vi "Recast Device.vi"(8 "error in":errorcluster, 11 "AlicatCommBank in":refnum<class "AlicatCommBank.lvclass">) -> (0 "error out":errorcluster, 3 "AlicatCommBank out":refnum<class "AlicatCommBank.lvclass">)   [LabVIEW 2015, in "Alicat.lvlib" / "AlicatCommBank.lvclass"]
doc: "This VI takes the Model number data and uses it to correctly cast the device types. Use this in conjunction with the Read Models VI to ensure that the model numbers are properly read in first. \n\nAlso, check register 20 - if the value is greater than 32768, then the controller is set up for back pressure control. In this case, we do not want to use the manufacturing data (since that will only tell the program the FS flow rate). Rather, use the original programatic input. If the input at config time is not correct, then the output will not scale correctly."
uses:
  AlicatCommBank.lvclass
  AlicatCommBank.lvclass/AlicatCommBank.ctl
  M/M.lvclass
  VC/Alicat_VC.lvclass
  V/V.lvclass
  P/P.lvclass
  MC/Alicat_MC.lvclass
  Alicat.lvclass
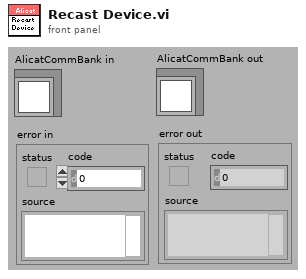
[diagram p1: front panel]
types:
  T1 = typedef "Alicat.lvlib/Alicat.lvclass/CtlSetup.ctl" = cluster{"Name":string, "Address":string, "fullScale":dbl, "Gas":T2}
  T2 = typedef "Alicat.lvlib/Alicat.lvclass/Gas.ctl" = enum16{"Air", "Ar", "CH4", "CO", "CO2", "C2H6", "H2", "He", "N2", "NO", "Ne", "O2", "C3H8", "n-C4H10", "C2H2", "C2H4", "i-C2H10", "Kr", "Xe"}
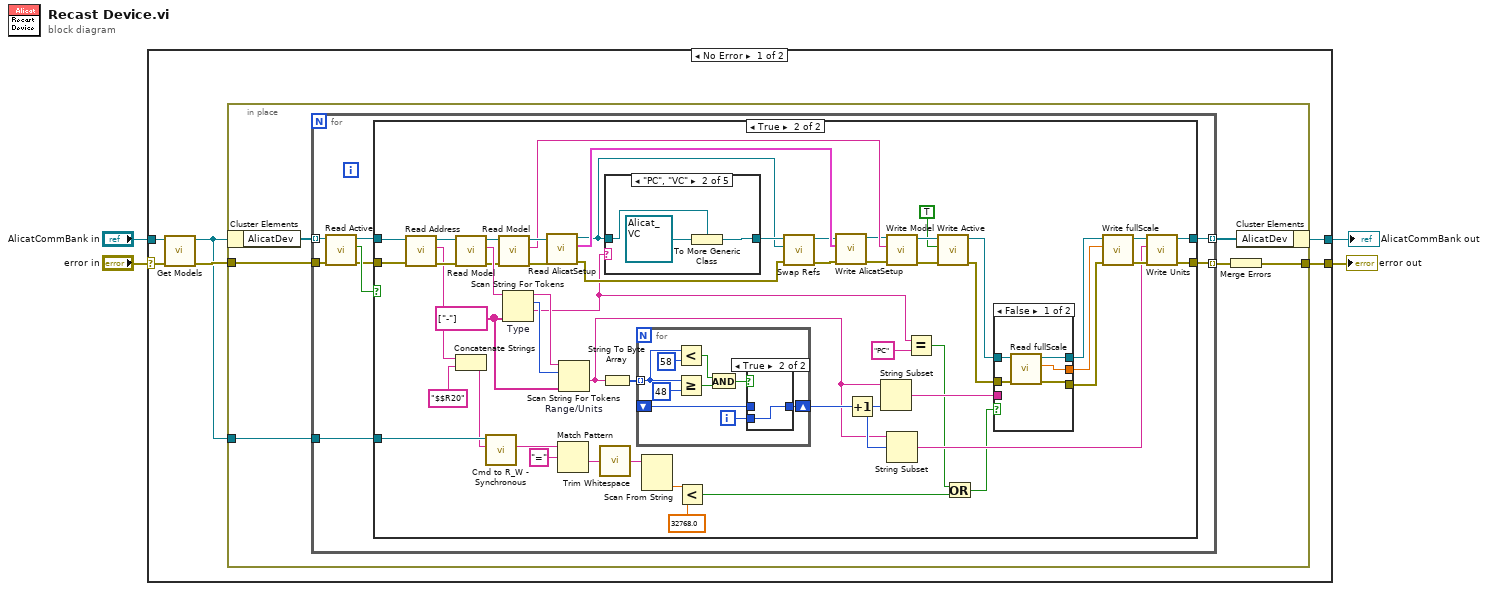
[diagram p0: block diagram]
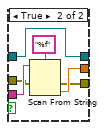
[diagram p3: hidden frame]
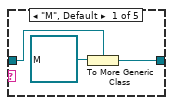
[diagram p5: hidden frame]
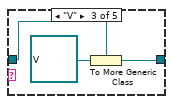
[diagram p6: hidden frame]
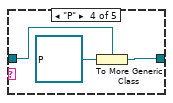
[diagram p7: hidden frame]
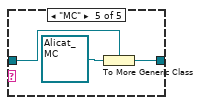
[diagram p8: hidden frame]
diagram:
  n1 = case shown="No Error" "error in" {
    selector: "error in" -> [w8 w119]
    tunnel: [w7 w119] -> w3
    tunnel: [w6 w118] -> w1
    tunnel: "AlicatCommBank in" -> [w10 w118]
    frame No Error {
      n2 = call "Get Models.vi"("error in"=w8, "AlicatCommBank in"=w10) -> ("error out"=w9:errorcluster, "AlicatCommBank out"=w5:refnum<class "AlicatCommBank.lvclass">)  [unwired: 8 in]
      n3 = in-place {
        in-place-border: w9 -> [w16]
        in-place-border: [w12] -> w7
        in-place-border: w5 -> [w11]
        n4 = in-place-cluster #1(w5) -> ("AlicatDev"=w15:refnum<class "Alicat.lvclass">[])
        n5 = for {
          tunnel: w15 -> [w21] mode=indexing
          tunnel: [w24] -> w14 mode=indexing
          tunnel: w16 -> [w20]
          tunnel: [w23] -> w13 mode=indexing
          tunnel: w11 -> [w22]
          n6 = call "Read Active.vi"("error in"=w20, "Alicat in"=w21) -> ("error out"=w17:errorcluster, "Active?"=w19:bool, "Alicat out"=w18:refnum<class "Alicat.lvclass">)  [unwired: 7 in]
          n7 = case shown="True" w19 {
            tunnel: [w26 w67] -> w24
            tunnel: [w25 w66] -> w23
            tunnel: w22 -> [_ w55]
            tunnel: w18 -> [w26 w38]
            tunnel: w17 -> [w25 w39]
            frame False {
            }
            frame True {
              w78 = string[] ["-"] ("operators (none)")
              n8 = call "Read Address.vi"("error in"=w39, "Alicat in"=w38) -> ("error out"=w56:errorcluster, "Address"=w54:string, "Alicat out"=w57:refnum<class "Alicat.lvclass">)  [unwired: 7 in]
              n9 = call "Read Model.vi"("error in (no error)"=w56, "Alicat in"=w57) -> ("error out"=w64:errorcluster, "Model"=w80:string, "Alicat out"=w65:refnum<class "Alicat.lvclass">)  [unwired: 7 in]
              n10 = Concatenate Strings(w54, "$$R20" ("string")) -> (w52:string)
              n11 = call-dynamic "Cmd to R_W - Synchronous.vi"("write buffer"=w52, "Serial IO in"=w55) -> ("read buffer"=w51:string)  [unwired: 7 in, 2 out]
              n12 = call "Read Model.vi"("error in (no error)"=w64, "Alicat in"=w65) -> ("error out"=w62:errorcluster, "Model"=w61:string, "Alicat out"=w63:refnum<class "Alicat.lvclass">)  [unwired: 7 in]
              n13 = Scan String For Tokens "Type"(6:w78, 9:w80) -> (1:w27:string, 2:w79:i32, 3:w31:string)  [unwired: 1 in, 4 out]
              n14 = call "Read AlicatSetup.vi"("error in (no error)"=w62, "Alicat in"=w63) -> ("error out"=w43:errorcluster, "AlicatSetup"=w59:T1, "Alicat out"=w40:refnum<class "Alicat.lvclass">)  [unwired: 7 in]
              n15 = Match Pattern(string=w51, regular expression="=") -> (after substring=w49:string)  [unwired: 1 in, 3 out]
              n16 = Scan String For Tokens "Range/Units"(6:w78, 8:w79, 9:w31) -> (1:w69:string)  [unwired: 6 out]
              n17 = call <vilib>:"Trim Whitespace.vi"("string"=w49) -> ("trimmed string"=w48:string)  [unwired: 1 in]
              n18 = String To Byte Array(string=w69) -> (unsigned byte array=w77:u8[])
              n19 = case shown="\"PC\", \"VC\"" w27 {
                tunnel: w40 -> [w103 w106 w109 w113 w115]
                tunnel: [w105 w108 w111 w114 w117] -> w44
                frame "M", Default {
                  n20 = To More Generic Class(target class=w103, reference=refnum<class "M.lvclass"> refnum ("M.lvclass")) -> (generic class reference=w105:refnum<class "Alicat.lvclass">)
                }
                frame "PC", "VC" {
                  n21 = To More Generic Class(target class=w106, reference=refnum<class "Alicat_VC.lvclass"> refnum ("Alicat_VC.lvclass")) -> (generic class reference=w108:refnum<class "Alicat.lvclass">)
                }
                frame "V" {
                  n22 = To More Generic Class(target class=w109, reference=refnum<class "V.lvclass"> refnum ("V.lvclass")) -> (generic class reference=w111:refnum<class "Alicat.lvclass">)
                }
                frame "P" {
                  n23 = To More Generic Class(target class=w113, reference=refnum<class "P.lvclass"> refnum ("Alicat_P.lvclass")) -> (generic class reference=w114:refnum<class "Alicat.lvclass">)
                }
                frame "MC" {
                  n24 = To More Generic Class(target class=w115, reference=refnum<class "Alicat_MC.lvclass"> refnum ("Alicat_MC.lvclass")) -> (generic class reference=w117:refnum<class "Alicat.lvclass">)
                }
              }
              n25 = for {
                tunnel: w77 -> [w95] mode=indexing
                shift-right: [w99] -> w75
                shift-left: _ -> [w92]
                i -> [w100]
                n26 = Less?(x=w95, y=u8 58) -> (x < y?=w97:bool)
                n27 = Greater Or Equal?(x=w95, y=u8 48) -> (x >= y?=w96:bool)
                n28 = And(x=w97, y=w96) -> (x .and. y?=w93:bool)
                n29 = case shown="True" w93 {
                  tunnel: w100 -> [_ w102]
                  tunnel: [w101 w102] -> w99
                  tunnel: w92 -> [w101 _]
                  frame False {
                  }
                  frame True {
                  }
                }
              }
              n30 = Scan From String(input string=w48) -> (output 1=w47:dbl)  [unwired: 4 in, 3 out]
              n31 = Less?(x=w47, y=32768.0) -> (x < y?=w32:bool)
              n32 = call-dynamic "Swap Refs.vi"("error in (no error)"=w43, "Old Ref"=w40, "New Ref"=w44) -> ("error out"=w42:errorcluster, "Alicat out"=w41:refnum<class "Alicat.lvclass">)  [unwired: 7 in]
              n33 = call "Write AlicatSetup.vi"("error in"=w42, "AlicatSetup"=w59, "Alicat in"=w41) -> ("error out"=w58:errorcluster, "Alicat out"=w60:refnum<class "Alicat.lvclass">)  [unwired: 7 in]
              n34 = Increment(x=w75) -> (x+1=w74:i32)
              n35 = String Subset(string=w69, length (rest)=w74) -> (substring=w76:string)  [unwired: 1 in]
              n36 = call "Write Model.vi"("error in"=w58, "Model"=w61, "Alicat in"=w60) -> ("error out"=w36:errorcluster, "Alicat out"=w37:refnum<class "Alicat.lvclass">)  [unwired: 7 in]
              n37 = String Subset(string=w69, offset (0)=w74) -> (substring=w70:string)  [unwired: 1 in]
              n38 = Equal?(x=w27, y="PC") -> (x = y?=w29:bool)
              n39 = call "Write Active.vi"("error in"=w36, "Active?"=TRUE, "Alicat in"=w37) -> ("error out"=w34:errorcluster, "Alicat out"=w35:refnum<class "Alicat.lvclass">)  [unwired: 7 in]
              n40 = Or(x=w29, y=w32) -> (x .or. y?=w28:bool)
              n41 = case shown="False" w28 {
                tunnel: w76 -> [_ w91]
                tunnel: [w81 w89] -> w71
                tunnel: [w83 w88] -> w68
                tunnel: w34 -> [w84 w87]
                tunnel: w35 -> [w85 w86]
                tunnel: [w82 w86] -> w45
                frame False {
                  n42 = call "Read fullScale.vi"("error in (no error)"=w84, "Alicat in"=w85) -> ("error out"=w83:errorcluster, "fullScale"=w81:dbl, "Alicat out"=w82:refnum<class "Alicat.lvclass">)  [unwired: 7 in]
                }
                frame True {
                  n43 = Scan From String(format string="%f", input string=w91, error in=w87) -> (error out=w88:errorcluster, output 1=w89:dbl)  [unwired: 2 in, 2 out]
                }
              }
              n44 = call "Write fullScale.vi"("error in (no error)"=w68, "fullScale"=w71, "Alicat in"=w45) -> ("error out"=w72:errorcluster, "Alicat out"=w73:refnum<class "Alicat.lvclass">)  [unwired: 7 in]
              n45 = call "Write Units.vi"("error in (no error)"=w72, "Units"=w70, "Alicat in"=w73) -> ("error out"=w66:errorcluster, "Alicat out"=w67:refnum<class "Alicat.lvclass">)  [unwired: 7 in]
            }
          }
        }
        n46 = Merge Errors(w13) -> (w12:errorcluster)
        n47 = in-place-cluster #1("AlicatDev"=w14) -> (w6:refnum<class "AlicatCommBank.lvclass">)
      }
    }
    frame Error {
    }
  }
  "error out" <- w3
  "AlicatCommBank out" <- w1
